vi "Delete From Array.vi"() -> ()   [LabVIEW 2014]
panel:
  out "已删除的部分":dbl[][](array[numeric])
  out "已删除的部分":dbl[](array[numeric])
  out "输出二维数组":dbl[][](array[numeric])
  out "输出一维数组":dbl[](array[numeric])
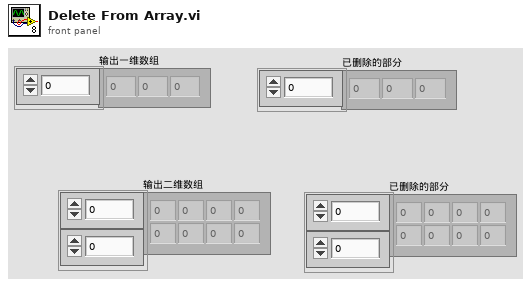
[diagram p1: front panel]
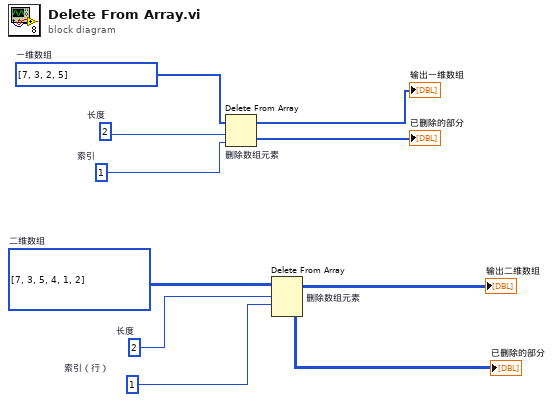
[diagram p0: block diagram]
diagram:
  w2 = 1  # 索引（行）
  w3 = 2  # 长度
  w5 = 1  # 索引
  w6 = 2  # 长度
  w8 = i32[][] [[7, 3, 5], [4, 1, 2]]  # 二维数组
  w10 = i32[] [7, 3, 2, 5]  # 一维数组
  n1 = Delete From Array "删除数组元素"(array=w10, length=w6, index=w5) -> (deleted portion=→"已删除的部分":i32[], array with subset deleted=→"输出一维数组":i32[])
  n2 = Delete From Array "删除数组元素"(array=w8, length=w3, index (row)=w2) -> (deleted portion=→"已删除的部分":i32[][], array with subset deleted=→"输出二维数组":i32[][])  [unwired: 1 in]
